vi "Get Date Timestamp.vi"(8 "error in (no error)":errorcluster) -> (0 "error out":errorcluster, 3 "current time":timestamp)   [LabVIEW 2015]
doc: "This VI might seem like overkill, however, the regular date/time VI does not have error terminals!"
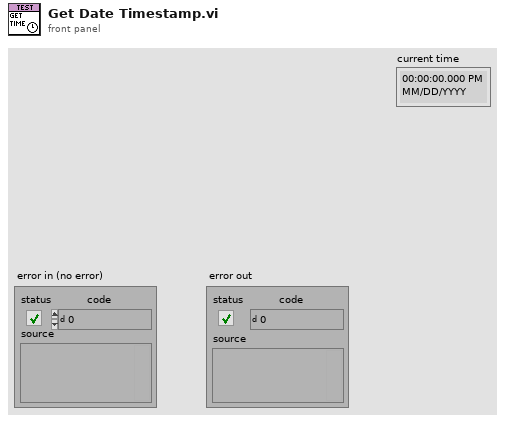
[diagram p1: front panel]
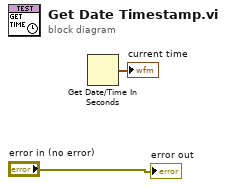
[diagram p0: block diagram]
diagram:
  n1 = Get Date/Time In Seconds() -> (seconds since 1Jan1904=→"current time":timestamp)
  "error out" <- "error in (no error)"
